vi "InsertNodes.vi"(6 "Insert Search":T1={"LLSearch in"=refnum, "InsertIfEmpty"=FALSE, "Insert After"=FALSE, "InsertIfNotFound"=TRUE}, 8 "error in (no error)":errorcluster, 9 "position":T2=enum."Back", 10 "ToInsert":refnum<data-value>, 11 "LinkedList in":refnum<class "LinkedList.lvclass">) -> (0 "error out":errorcluster, 1 "ignored":bool, 3 "LinkedList out":refnum<class "LinkedList.lvclass">)   [LabVIEW 2009, in "LinkedList.lvclass"]
uses:
  LinkedList.lvclass
  position.ctl
  LLNode/LLNode.lvclass
  InsertSearch.ctl
  LLSearch/LLSearch.lvclass
  Node/Node.lvclass
  Structure/Structure.lvclass
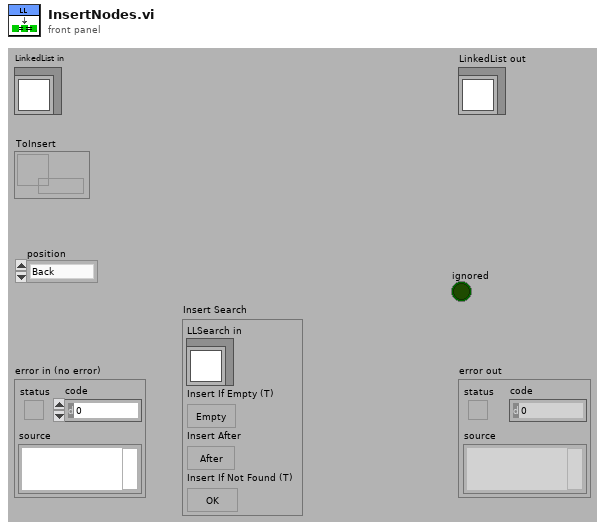
[diagram p1: front panel]
types:
  T1 = typedef "LinkedList.lvclass/InsertSearch.ctl" = cluster{"LLSearch in":refnum<class "LLSearch.lvclass">, "InsertIfEmpty":bool, "Insert After":bool, "InsertIfNotFound":bool}
  T2 = typedef "LinkedList.lvclass/position.ctl" = enum16{"Front", "Back", "Search"}
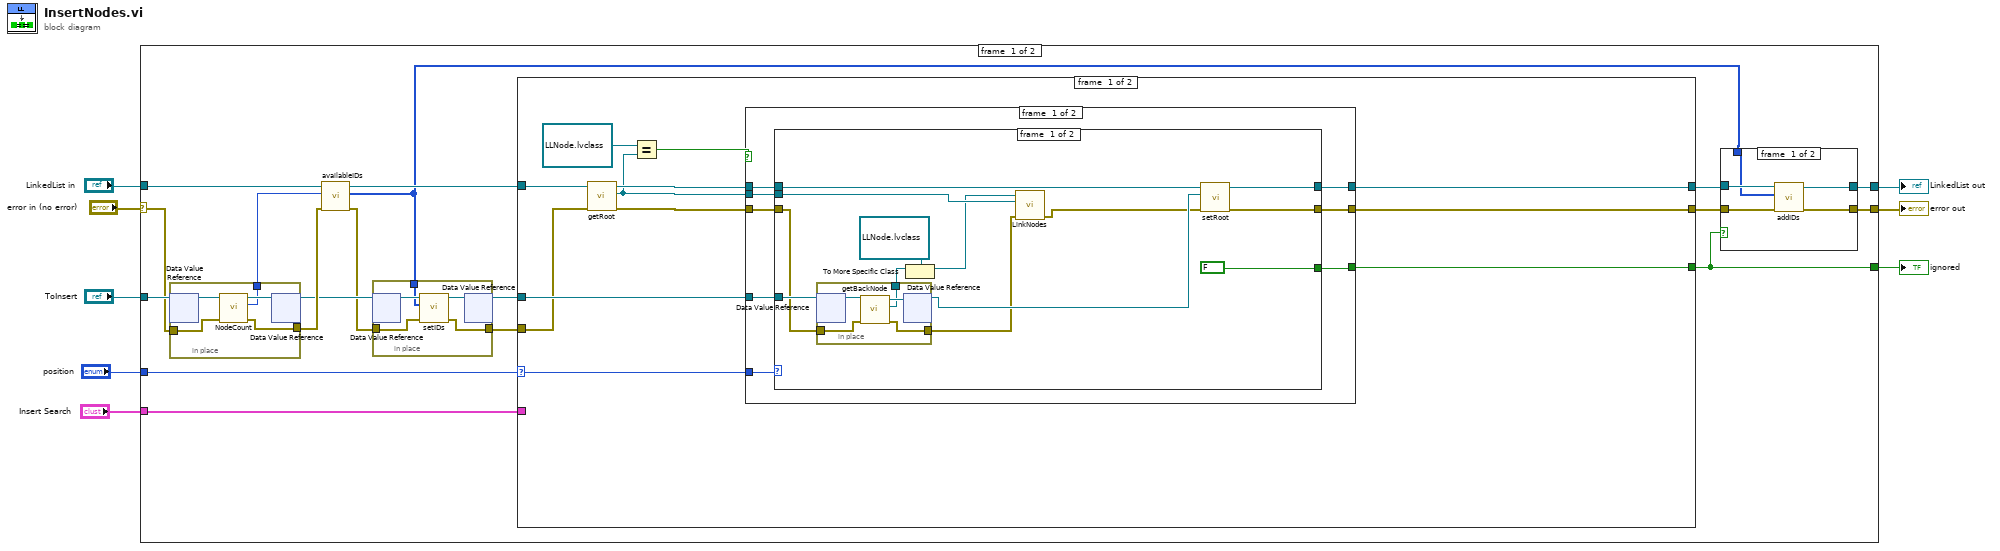
[diagram p0: block diagram]
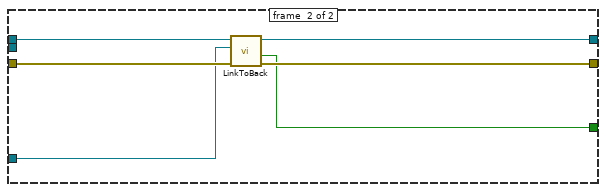
[diagram p3: hidden frame]
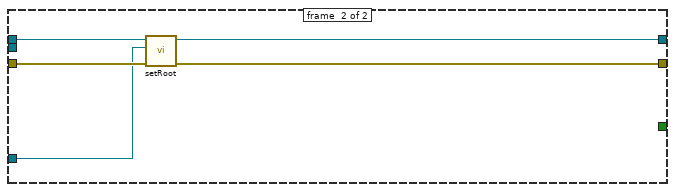
[diagram p4: hidden frame]
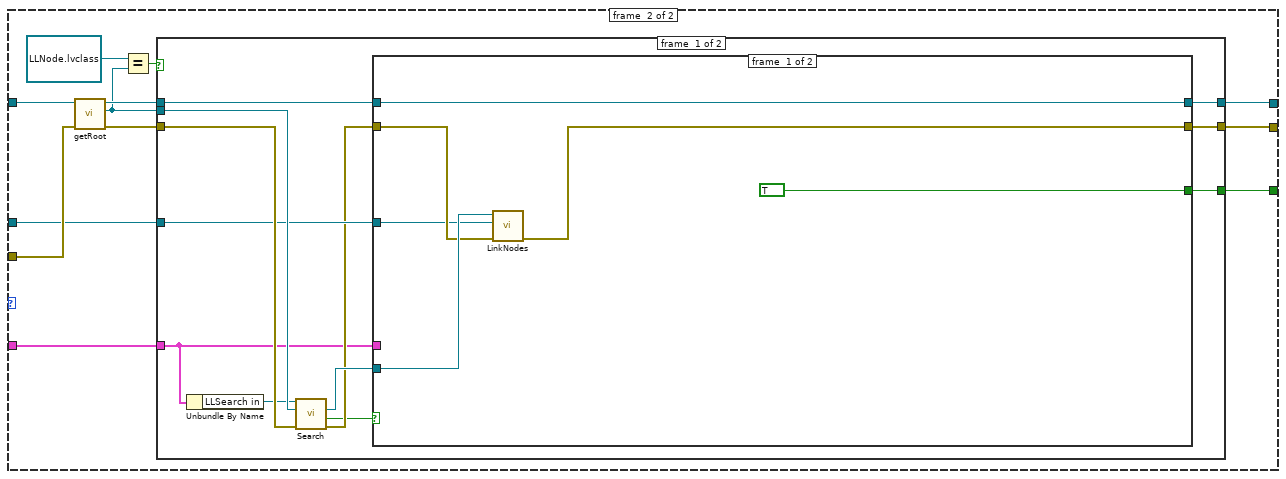
[diagram p5: hidden frame]
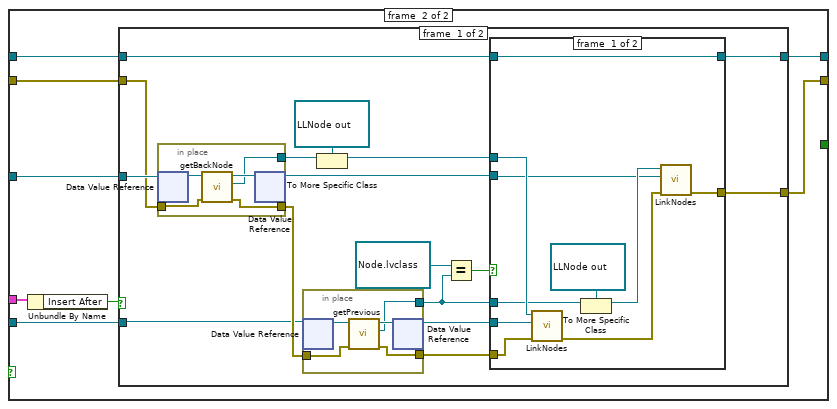
[diagram p6: hidden frame]
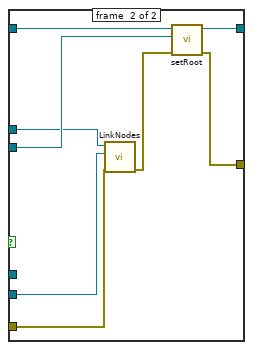
[diagram p7: hidden frame]
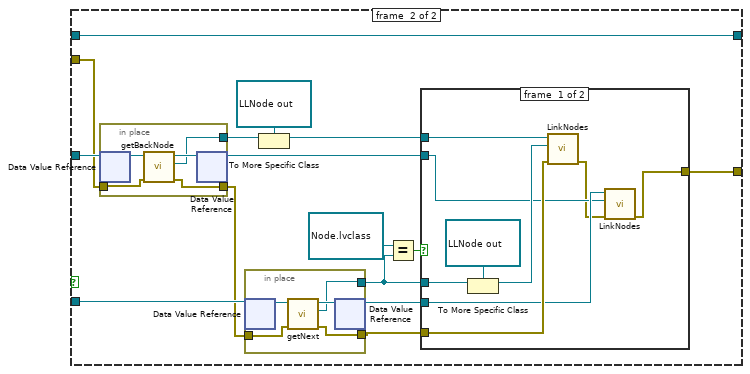
[diagram p8: hidden frame]
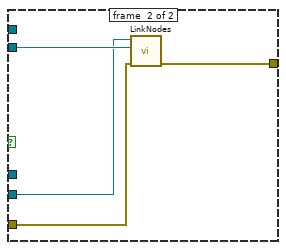
[diagram p9: hidden frame]
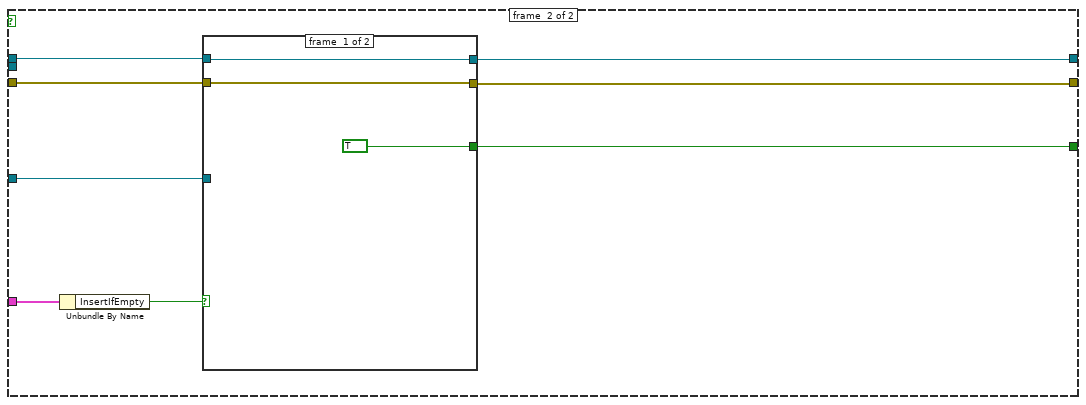
[diagram p10: hidden frame]
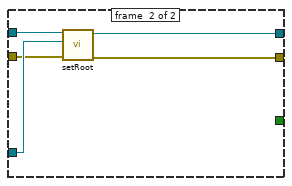
[diagram p11: hidden frame]
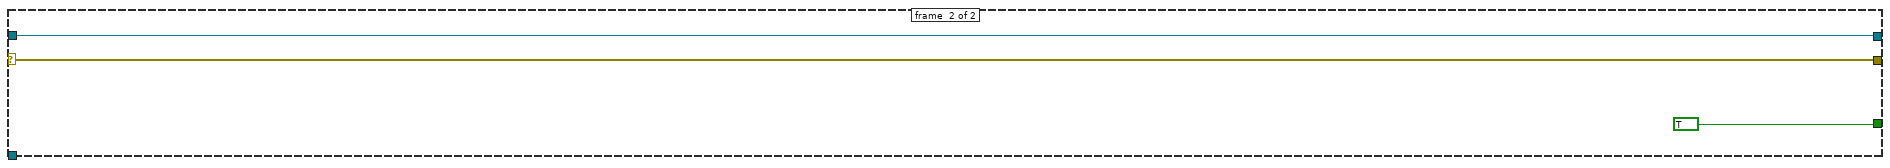
[diagram p12: hidden frame]
diagram:
  n1 = case shown="No Error" "error in (no error)" {
    selector: "error in (no error)" -> [w24 w231]
    tunnel: [w12 w231] -> w7
    tunnel: [w13 w230] -> w6
    tunnel: "LinkedList in" -> [w23 w230]
    tunnel: "ToInsert" -> [w25 _]
    tunnel: "position" -> [w26 _]
    tunnel: [w15 TRUE] -> w2
    tunnel: "Insert Search" -> [w9 _]
    frame #0 {
      n2 = in-place {
        in-place-border: w24 -> [w41]
        in-place-border: [w40] -> w21
        in-place-border: [w39] -> w20
        n3 = in-place-dvr #1(w25) -> (w43:refnum<class "LLNode.lvclass">)  [unwired: 1 out]
        n4 = call "NodeCount.vi"("error in (no error)"=w41, "LLNode in"=w43) -> ("error out"=w40:errorcluster, "count out"=w39:u32, "LLNode out"=w42:refnum<class "LLNode.lvclass">)  [unwired: 7 in]
        n5 = in-place-dvr #1(w42) -> (w18:refnum<data-value>)  [unwired: 1 out]
      }
      n6 = call "availableIDs.vi"("error in (no error)"=w21, "NumberOfIDs"=w20, "Structure in"=w23) -> ("error out"=w17:errorcluster, "IDs"=w10:u32[], "Structure out"=w22:refnum<class "LinkedList.lvclass">)  [unwired: 6 in]
      n7 = in-place {
        in-place-border: w10 -> [w36]
        in-place-border: w17 -> [w35]
        in-place-border: [w34] -> w16
        n8 = in-place-dvr #2(w18) -> (w38:refnum<class "LLNode.lvclass">)  [unwired: 1 out]
        n9 = call "setIDs.vi"("error in (no error)"=w35, "IDs"=w36, "LLNode in"=w38) -> ("error out"=w34:errorcluster, "LLNode out"=w37:refnum<class "LLNode.lvclass">)  [unwired: 7 in]
        n10 = in-place-dvr #2(w37) -> (w19:refnum<data-value>)  [unwired: 1 out]
      }
      n11 = case shown="\"Search\"" w26 {
        selector: w26 -> [w50 _]
        tunnel: w22 -> [w47 w103]
        tunnel: [w45 w98] -> w14
        tunnel: [w44 w97] -> w11
        tunnel: [w49 w96] -> w15
        tunnel: w19 -> [w48 w93]
        tunnel: w16 -> [w46 w102]
        tunnel: w9 -> [_ w94]
        frame #0 {
          n12 = call "getRoot.vi"("error in (no error)"=w46, "LinkedList in"=w47) -> ("error out"=w53:errorcluster, "Root"=w51:refnum<data-value>, "LinkedList out"=w52:refnum<class "LinkedList.lvclass">)  [unwired: 7 in]
          n13 = Equal?(x=refnum<data-value> refnum, y=w51) -> (x = y?=w54:bool)
          n14 = case shown="True" w54 {
            tunnel: w53 -> [w62 w92]
            tunnel: w52 -> [w57 w91]
            tunnel: w48 -> [w60 w90]
            tunnel: [w56 w89] -> w45
            tunnel: w51 -> [w63 _]
            tunnel: [w61 w88] -> w44
            tunnel: w50 -> [w58 _]
            tunnel: [w59 _] -> w49
            frame #0 {
              n15 = case shown="\"Front\", Default" w58 {
                tunnel: w63 -> [w65 _]
                tunnel: w62 -> [w70 w86]
                tunnel: [w75 w85] -> w61
                tunnel: w60 -> [w73 w83]
                tunnel: [FALSE ("ignored") w82] -> w59
                tunnel: w57 -> [w76 w87]
                tunnel: [w74 w84] -> w56
                frame #0 {
                  n16 = in-place {
                    in-place-border: [w79] -> w72
                    in-place-border: w70 -> [w78]
                    in-place-border: [w77] -> w67
                    n17 = in-place-dvr #3(w73) -> (w81:refnum<class "LLNode.lvclass">)  [unwired: 1 out]
                    n18 = call "getBackNode.vi"("error in (no error)"=w78, "LLNode in"=w81) -> ("error out"=w77:errorcluster, "BackNode"=w79:refnum<data-value>, "LLNode out"=w80:refnum<class "LLNode.lvclass">)  [unwired: 7 in]
                    n19 = in-place-dvr #3(w80) -> (w68:refnum<data-value>)  [unwired: 1 out]
                  }
                  n20 = To More Specific Class(target class=refnum<data-value> refnum ("x"), reference=w72) -> (specific class reference=w64:refnum<data-value>)  [unwired: 1 in, 1 out]
                  n21 = call "LinkNodes.vi"("error in (no error)"=w67, "NextNode in"=w65, "PreviousNode in"=w64) -> ("error out"=w66:errorcluster)  [unwired: 6 in, 2 out]
                  n22 = call "setRoot.vi"("error in (no error)"=w66, "Root"=w68, "LinkedList in"=w76) -> ("error out"=w75:errorcluster, "LinkedList out"=w74:refnum<class "LinkedList.lvclass">)  [unwired: 7 in]
                }
                frame #1 {
                  n23 = call "LinkToBack.vi"("error in (no error)"=w86, "newBackNode"=w83, "LinkedList in"=w87) -> ("error out"=w85:errorcluster, "ignored"=w82:bool, "LinkedList out"=w84:refnum<class "LinkedList.lvclass">)  [unwired: 6 in]
                }
              }
            }
            frame #1 {
              n24 = call "setRoot.vi"("error in (no error)"=w92, "Root"=w90, "LinkedList in"=w91) -> ("error out"=w88:errorcluster, "LinkedList out"=w89:refnum<class "LinkedList.lvclass">)  [unwired: 7 in]
            }
          }
        }
        frame #1 {
          n25 = call "getRoot.vi"("error in (no error)"=w102, "LinkedList in"=w103) -> ("error out"=w99:errorcluster, "Root"=w95:refnum<data-value>, "LinkedList out"=w100:refnum<class "LinkedList.lvclass">)  [unwired: 7 in]
          n26 = Equal?(x=refnum<data-value> refnum, y=w95) -> (x = y?=w101:bool)
          n27 = case shown="False" w101 {
            tunnel: w100 -> [w106 w219]
            tunnel: w99 -> [w116 w216]
            tunnel: [w105 w214] -> w98
            tunnel: [w111 w215] -> w97
            tunnel: [w107 w213] -> w96
            tunnel: w95 -> [w115 _]
            tunnel: w94 -> [w108 w220]
            tunnel: w93 -> [w113 w217]
            frame #0 {
              n28 = Unbundle By Name(w108) -> ("LLSearch in"=w109:refnum<class "LLSearch.lvclass">)
              n29 = call "Search.vi"("error in (no error)"=w116, "LLNode in"=w115, "LLSearch in"=w109) -> ("error out"=w112:errorcluster, "found"=w110:bool, "LLNode out"=w114:refnum<data-value>)  [unwired: 5 in, 1 out]
              n30 = case shown="False" w110 {
                tunnel: w114 -> [w120 w126]
                tunnel: w113 -> [w118 w127]
                tunnel: w112 -> [w119 w128]
                tunnel: [w117 w125] -> w111
                tunnel: w108 -> [_ w130]
                tunnel: [TRUE _] -> w107
                tunnel: w106 -> [w121 w124]
                tunnel: [w121 w123] -> w105
                frame #0 {
                  n31 = call "LinkNodes.vi"("error in (no error)"=w119, "NextNode in"=w118, "PreviousNode in"=w120) -> ("error out"=w117:errorcluster)  [unwired: 6 in, 2 out]
                }
                frame #1 {
                  n32 = Unbundle By Name(w130) -> ("Insert After"=w129:bool)
                  n33 = case shown="False" w129 {
                    tunnel: w128 -> [w140 w186]
                    tunnel: w127 -> [w142 w189]
                    tunnel: w126 -> [w141 w185]
                    tunnel: [w133 w176] -> w125
                    tunnel: w124 -> [w132 w175]
                    tunnel: [w131 w175] -> w123
                    frame #0 {
                      n34 = in-place {
                        in-place-border: [w172] -> w145
                        in-place-border: w140 -> [w171]
                        in-place-border: [w170] -> w144
                        n35 = in-place-dvr #4(w142) -> (w174:refnum<class "LLNode.lvclass">)  [unwired: 1 out]
                        n36 = call "getBackNode.vi"("error in (no error)"=w171, "LLNode in"=w174) -> ("error out"=w170:errorcluster, "BackNode"=w172:refnum<data-value>, "LLNode out"=w173:refnum<class "LLNode.lvclass">)  [unwired: 7 in]
                        n37 = in-place-dvr #4(w173) -> (w138:refnum<data-value>)  [unwired: 1 out]
                      }
                      n38 = in-place {
                        in-place-border: [w167] -> w134
                        in-place-border: w144 -> [w166]
                        in-place-border: [w165] -> w135
                        n39 = in-place-dvr #5(w141) -> (w169:refnum<class "LLNode.lvclass">)  [unwired: 1 out]
                        n40 = call "getPrevious.vi"("error in (no error)"=w166, "LLNode in"=w169) -> ("error out"=w165:errorcluster, "previous"=w167:refnum<data-value>, "LLNode out"=w168:refnum<class "LLNode.lvclass">)  [unwired: 7 in]
                        n41 = in-place-dvr #5(w168) -> (w136:refnum<data-value>)  [unwired: 1 out]
                      }
                      n42 = To More Specific Class(target class=refnum<data-value> refnum ("ToInsert"), reference=w145) -> (specific class reference=w137:refnum<data-value>)  [unwired: 1 in, 1 out]
                      n43 = Equal?(x=refnum<data-value> refnum, y=w134) -> (x = y?=w139:bool)
                      n44 = case shown="False" w139 {
                        tunnel: w138 -> [w148 w162]
                        tunnel: w137 -> [w153 w160]
                        tunnel: w136 -> [w155 w161]
                        tunnel: w135 -> [w154 w159]
                        tunnel: w134 -> [w152 _]
                        tunnel: [w149 w157] -> w133
                        tunnel: w132 -> [w156 w164]
                        tunnel: [w156 w163] -> w131
                        frame #0 {
                          n45 = call "LinkNodes.vi"("error in (no error)"=w154, "NextNode in"=w155, "PreviousNode in"=w153) -> ("error out"=w147:errorcluster)  [unwired: 6 in, 2 out]
                          n46 = To More Specific Class(target class=refnum<data-value> refnum ("ToInsert"), reference=w152) -> (specific class reference=w150:refnum<data-value>)  [unwired: 1 in, 1 out]
                          n47 = call "LinkNodes.vi"("error in (no error)"=w147, "NextNode in"=w148, "PreviousNode in"=w150) -> ("error out"=w149:errorcluster)  [unwired: 6 in, 2 out]
                        }
                        frame #1 {
                          n48 = call "LinkNodes.vi"("error in (no error)"=w159, "NextNode in"=w161, "PreviousNode in"=w160) -> ("error out"=w158:errorcluster)  [unwired: 6 in, 2 out]
                          n49 = call "setRoot.vi"("error in (no error)"=w158, "Root"=w162, "LinkedList in"=w164) -> ("error out"=w157:errorcluster, "LinkedList out"=w163:refnum<class "LinkedList.lvclass">)  [unwired: 7 in]
                        }
                      }
                    }
                    frame #1 {
                      n50 = in-place {
                        in-place-border: [w210] -> w187
                        in-place-border: w186 -> [w209]
                        in-place-border: [w208] -> w184
                        n51 = in-place-dvr #6(w189) -> (w212:refnum<class "LLNode.lvclass">)  [unwired: 1 out]
                        n52 = call "getBackNode.vi"("error in (no error)"=w209, "LLNode in"=w212) -> ("error out"=w208:errorcluster, "BackNode"=w210:refnum<data-value>, "LLNode out"=w211:refnum<class "LLNode.lvclass">)  [unwired: 7 in]
                        n53 = in-place-dvr #6(w211) -> (w181:refnum<data-value>)  [unwired: 1 out]
                      }
                      n54 = in-place {
                        in-place-border: [w205] -> w179
                        in-place-border: w184 -> [w204]
                        in-place-border: [w203] -> w177
                        n55 = in-place-dvr #7(w185) -> (w207:refnum<class "LLNode.lvclass">)  [unwired: 1 out]
                        n56 = call "getNext.vi"("error in (no error)"=w204, "LLNode in"=w207) -> ("error out"=w203:errorcluster, "next"=w205:refnum<data-value>, "LLNode out"=w206:refnum<class "LLNode.lvclass">)  [unwired: 7 in]
                        n57 = in-place-dvr #7(w206) -> (w178:refnum<data-value>)  [unwired: 1 out]
                      }
                      n58 = To More Specific Class(target class=refnum<data-value> refnum ("ToInsert"), reference=w187) -> (specific class reference=w180:refnum<data-value>)  [unwired: 1 in, 1 out]
                      n59 = Equal?(x=refnum<data-value> refnum, y=w179) -> (x = y?=w182:bool)
                      n60 = case shown="True" w182 {
                        tunnel: w181 -> [w192 w202]
                        tunnel: w180 -> [w198 _]
                        tunnel: w179 -> [w197 _]
                        tunnel: w178 -> [w193 w201]
                        tunnel: w177 -> [w194 w200]
                        tunnel: [w190 w199] -> w176
                        frame #0 {
                          n61 = To More Specific Class(target class=refnum<data-value> refnum ("ToInsert"), reference=w197) -> (specific class reference=w195:refnum<data-value>)  [unwired: 1 in, 1 out]
                          n62 = call "LinkNodes.vi"("error in (no error)"=w194, "NextNode in"=w195, "PreviousNode in"=w198) -> ("error out"=w191:errorcluster)  [unwired: 6 in, 2 out]
                          n63 = call "LinkNodes.vi"("error in (no error)"=w191, "NextNode in"=w192, "PreviousNode in"=w193) -> ("error out"=w190:errorcluster)  [unwired: 6 in, 2 out]
                        }
                        frame #1 {
                          n64 = call "LinkNodes.vi"("error in (no error)"=w200, "NextNode in"=w202, "PreviousNode in"=w201) -> ("error out"=w199:errorcluster)  [unwired: 6 in, 2 out]
                        }
                      }
                    }
                  }
                }
              }
            }
            frame #1 {
              n65 = Unbundle By Name(w220) -> ("InsertIfEmpty"=w218:bool)
              n66 = case shown="True" w218 {
                tunnel: w219 -> [w221 w228]
                tunnel: w217 -> [_ w227]
                tunnel: w216 -> [w222 w226]
                tunnel: [w222 w225] -> w215
                tunnel: [w221 w224] -> w214
                tunnel: [TRUE _] -> w213
                frame #0 {
                }
                frame #1 {
                  n67 = call "setRoot.vi"("error in (no error)"=w226, "Root"=w227, "LinkedList in"=w228) -> ("error out"=w225:errorcluster, "LinkedList out"=w224:refnum<class "LinkedList.lvclass">)  [unwired: 7 in]
                }
              }
            }
          }
        }
      }
      n68 = case shown="False" w15 {
        tunnel: w14 -> [w31 w33]
        tunnel: [w30 w33] -> w13
        tunnel: w11 -> [w29 w32]
        tunnel: [w28 w32] -> w12
        tunnel: w10 -> [w27 _]
        frame #0 {
          n69 = call "addIDs.vi"("error in (no error)"=w29, "new IDs"=w27, "Structure in"=w31) -> ("error out"=w28:errorcluster, "Structure out"=w30:refnum<class "LinkedList.lvclass">)  [unwired: 7 in]
        }
        frame #1 {
        }
      }
    }
    frame #1 {
    }
  }
  "error out" <- w7
  "LinkedList out" <- w6
  "ignored" <- w2
